vi "Read Name Lookup Table (GUID should return Name).vi"(11 "ServerListener in":refnum<class "ServerListener.lvclass">) -> (2 "Name Lookup Table (GUID should return Name)":variant, 3 "ServerListener out":refnum<class "ServerListener.lvclass">)   [LabVIEW 2016, in "ServerListener.lvlib" / "ServerListener.lvclass"]
uses:
  ServerListener.lvclass
  ServerListener.lvclass/ServerListener.ctl
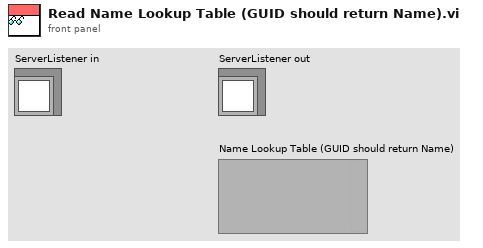
[diagram p1: front panel]
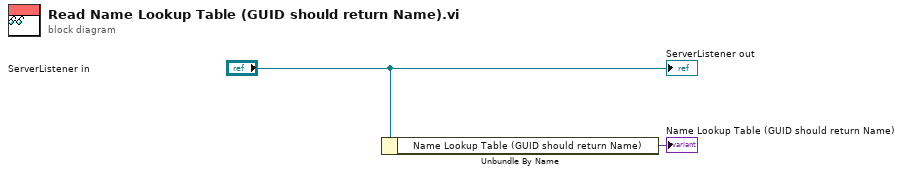
[diagram p0: block diagram]
diagram:
  n1 = Unbundle By Name("ServerListener in") -> ("Name Lookup Table (GUID should return Name)"=→"Name Lookup Table (GUID should return Name)":variant)
  "ServerListener out" <- "ServerListener in"
